vi "Set Current Iteration.vi"(9 "iteration valid (T)":bool=TRUE, 10 "iteration":u64=1, 11 "Transfer Group in":refnum<class "Transfer Group.lvclass">) -> (3 "Transfer Group out":refnum<class "Transfer Group.lvclass">)   [LabVIEW 2019, in "DSF Core.lvlib" / "Transfer Group.lvclass"]
uses:
  Transfer Group.lvclass
  Transfer Group.lvclass/Transfer Group.ctl
  Timing/Timing.lvclass/Timing.ctl
  Timing/Timing.lvclass
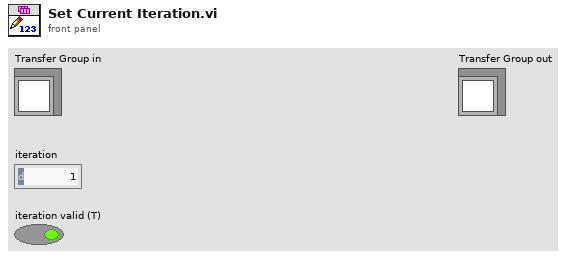
[diagram p1: front panel]
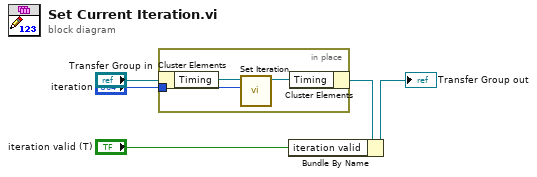
[diagram p0: block diagram]
diagram:
  n1 = in-place {
    in-place-border: "iteration" -> [w6]
    n2 = in-place-cluster #1("Transfer Group in") -> ("Timing"=w8:refnum<class "Timing.lvclass">)
    n3 = call "Set Iteration.vi"("Iteration"=w6, "Timing in"=w8) -> ("Timing out"=w7:refnum<class "Timing.lvclass">)  [unwired: 9 in]
    n4 = in-place-cluster #1("Timing"=w7) -> (w3:refnum<class "Transfer Group.lvclass">)
  }
  n5 = Bundle By Name(cluster=w3, "iteration valid"="iteration valid (T)") -> (→"Transfer Group out":refnum<class "Transfer Group.lvclass">)
